vi "CTOparamValArray.vi"(0 "zIdx":i32, 5 "initPos (mm)":dbl, 7 "finPos (mm)":dbl, 9 "stepSize (mm)":dbl, 11 "initTrigPos (mm)":dbl) -> (8 "CTOparamValArray":string[](array[string]))   [LabVIEW 2015]
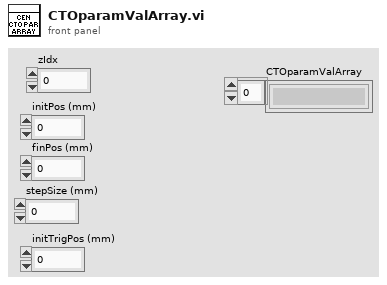
[diagram p1: front panel]
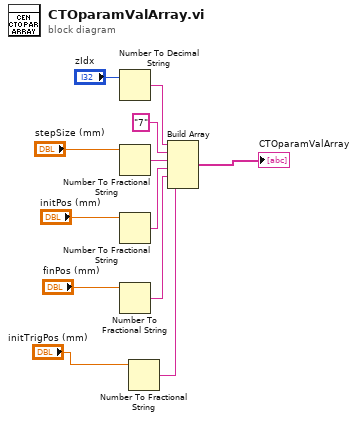
[diagram p0: block diagram]
diagram:
  n1 = Number To Decimal String(number="zIdx") -> (decimal integer string=w12:string)  [unwired: 1 in]
  n2 = Number To Fractional String(number="stepSize (mm)") -> (F-format string=w10:string)  [unwired: 3 in]
  n3 = Number To Fractional String(number="initPos (mm)") -> (F-format string=w9:string)  [unwired: 3 in]
  n4 = Number To Fractional String(number="finPos (mm)") -> (F-format string=w8:string)  [unwired: 3 in]
  n5 = Number To Fractional String(number="initTrigPos (mm)") -> (F-format string=w1:string)  [unwired: 3 in]
  n6 = Build Array(w12, "7" ("element"), w10, w9, w8, w1) -> (→"CTOparamValArray":string[])
